vi "hinzufügen zu playlist.vi"(1 "letzte zeile 3":i32, 4 "Numerisches Element":i32, 5 "String":string, 6 "String 2":string, 7 "Referenz 3":refnum<vi>, 8 "filename without extension":string, 9 "Referenz 2":refnum<vi>, 10 "Referenz":refnum<vi>) -> (0 "letzte zeile 2":i32, 2 "Numerisches Element 2":i32, 3 "Zeilezumeinfügen":i32=4)   [LabVIEW 2010]
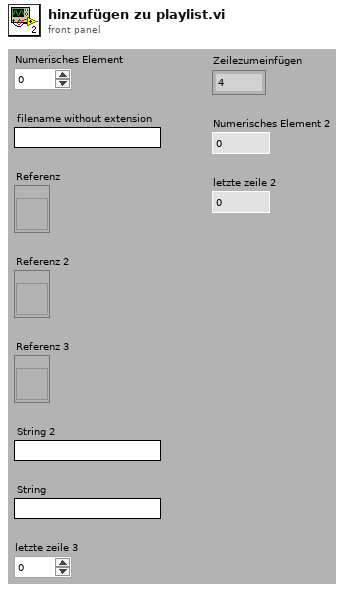
[diagram p1: front panel]
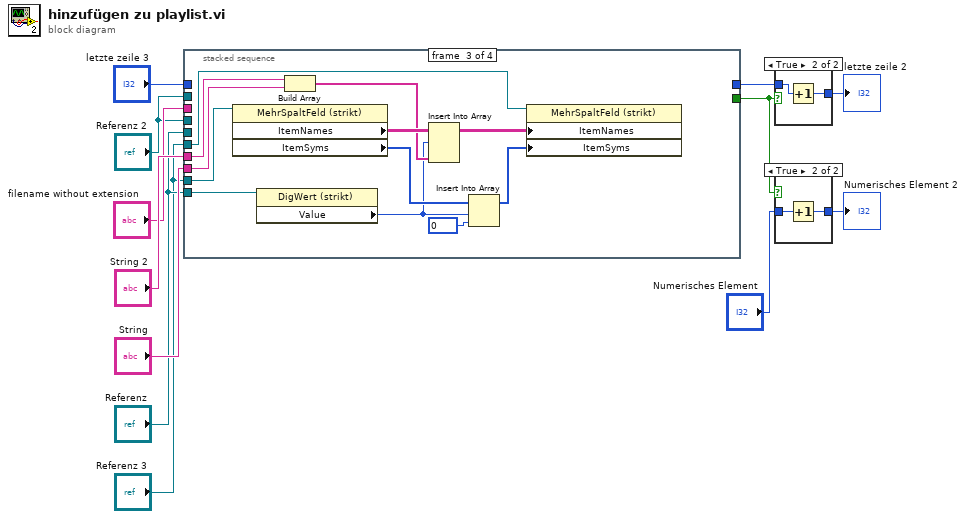
[diagram p0: block diagram]
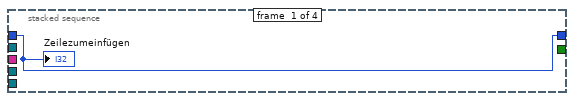
[diagram p2: hidden frame]
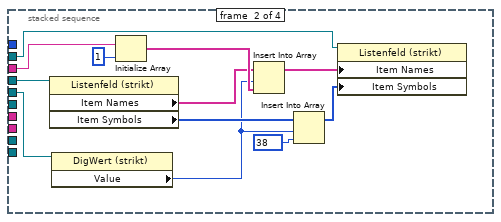
[diagram p3: hidden frame]
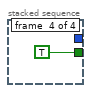
[diagram p4: hidden frame]
diagram:
  n1 = stacked-sequence {
    tunnel: [_ _ _ TRUE] -> w10
    tunnel: "filename without extension" -> [_ w23 _ _]
    tunnel: "String 2" -> [_ _ w35 _]
    tunnel: "String" -> [_ _ w34 _]
    tunnel: "letzte zeile 3" -> [w13 _ _ _]
    tunnel: [w13 _ _ _] -> w11
    tunnel: "Referenz" -> [_ w16 _ _]
    tunnel: "Referenz 2" -> [_ w15 _ _]
    tunnel: "Referenz 2" -> [_ w14 _ _]
    tunnel: "Referenz" -> [_ _ w28 _]
    tunnel: "Referenz 3" -> [_ _ w27 _]
    tunnel: "Referenz 3" -> [_ _ w26 _]
    frame #0 {
      "Zeilezumeinfügen" <- w13
    }
    frame #1 {
      n2 = property on="Eigenschaftsknoten" class="Listenfeld (strikt)"(reference=w15) -> ("Item Names"=w22:string[], "Item Symbols"=w19:i32[])  [unwired: 1 in, 2 out]
      n3 = property class="DigWert (strikt)"(reference=w16) -> ("Value"=w18:i32)  [unwired: 1 in, 2 out]
      n4 = Initialize Array(w23, 1 ("Dimension")) -> (w24:string[])
      n5 = Insert Into Array(array=w22, index=w18, new element=w24) -> (w21:string[])
      n6 = Insert Into Array(array=w19, index=w18, new element=38) -> (w20:i32[])
      n7 = property on="Eigenschaftsknoten" class="Listenfeld (strikt)"(reference=w14, "Item Names"=w21, "Item Symbols"=w20) -> ()  [unwired: 1 in, 2 out]
    }
    frame #2 {
      n8 = property on="Eigenschaftsknoten" class="MehrSpaltFeld (strikt)"(reference=w27) -> ("ItemNames"=w37:string[][], "ItemSyms"=w31:i32[])  [unwired: 1 in, 2 out]
      n9 = property class="DigWert (strikt)"(reference=w28) -> ("Value"=w30:i32)  [unwired: 1 in, 2 out]
      n10 = Build Array(w35, w34) -> (w36:string[])
      n11 = Insert Into Array(array=w37, index (row)=w30, new element=w36) -> (w33:string[][])  [unwired: 1 in]
      n12 = Insert Into Array(array=w31, index=w30, new element=0) -> (w29:i32[])
      n13 = property on="Eigenschaftsknoten" class="MehrSpaltFeld (strikt)"(reference=w26, "ItemNames"=w33, "ItemSyms"=w29) -> ()  [unwired: 1 in, 2 out]
    }
    frame #3 {
    }
  }
  n14 = case shown="TRUE" w10 {
    tunnel: w11 -> [w39 w41]
    tunnel: [w39 w40] -> w12
    frame False {
    }
    frame True {
      n15 = Increment(x=w41) -> (x+1=w40:i32)
    }
  }
  "letzte zeile 2" <- w12
  n16 = case shown="TRUE" w10 {
    tunnel: "Numerisches Element" -> [w42 w44]
    tunnel: [w42 w43] -> w4
    frame False {
    }
    frame True {
      n17 = Increment(x=w44) -> (x+1=w43:i32)
    }
  }
  "Numerisches Element 2" <- w4
